vi "Send dashboard control.vi"(7 "timeout":i32=1000, 8 "error in":errorcluster, 10 "Dashboard Control":T1={"Tractive System"=TRUE, "RTD"=TRUE, "AMS error"=TRUE, "IMD error"=TRUE, "Low Voltage"=0.0, "High Voltage"=0.0} {"High Voltage" scale=0.0..10.0; "Low Voltage" scale=0.0..10.0}, 11 "CAN Session In":T2) -> (0 "error out":errorcluster, 3 "CAN Session Out":T2)   [LabVIEW 2016]
uses:
  Program Files (x86)/National Instruments/LabVIEW 2016/examples/robotics/EPOS2 CANOpen Driver/Low Level VIs/Typedefs/CAN Refnum.ctl
  Program Files (x86)/National Instruments/LabVIEW 2016/examples/robotics/EPOS2 CANOpen Driver/Low Level VIs/Typedefs/CAN Session Pointer.ctl
  Program Files (x86)/National Instruments/LabVIEW 2016/examples/robotics/EPOS2 CANOpen Driver/Low Level VIs/Typedefs/CAN Communication References.ctl
  Program Files (x86)/National Instruments/LabVIEW 2016/examples/robotics/EPOS2 CANOpen Driver/Low Level VIs/Typedefs/kill process notifier array.ctl
  Program Files (x86)/National Instruments/LabVIEW 2016/examples/robotics/EPOS2 CANOpen Driver/Low Level VIs/Typedefs/Write Queue.ctl
  Program Files (x86)/National Instruments/LabVIEW 2016/examples/robotics/EPOS2 CANOpen Driver/Low Level VIs/Typedefs/FPGA CAN Frame Cluster.ctl
  Dashboard Control.ctl
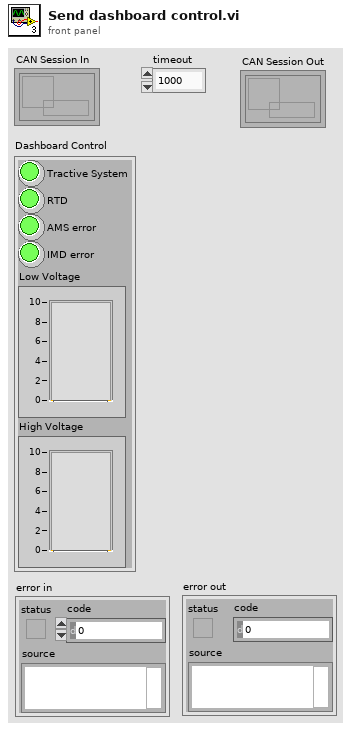
[diagram p1: front panel]
types:
  T1 = typedef "Dashboard Control.ctl" = cluster{"Tractive System":bool, "RTD":bool, "AMS error":bool, "IMD error":bool, "Low Voltage":dbl, "High Voltage":dbl}
  T2 = typedef "CAN Refnum.ctl" = refnum<k1>
  T3 = typedef "FPGA CAN Frame Cluster.ctl" = cluster{"Timestamp":u64, "Identifier":u32, "Type":u8, "InfoA":u8, "InfoB":u8, "DataLength":u8, "Data":u8[]}
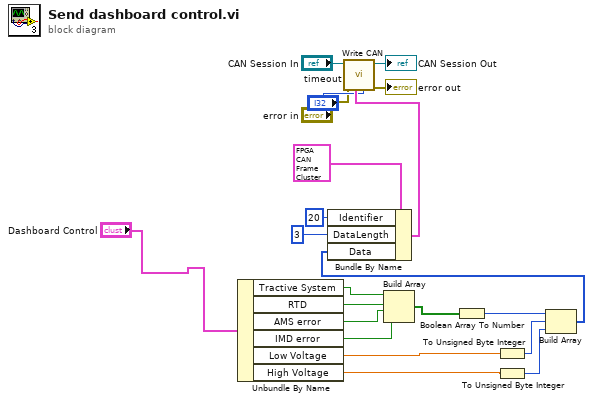
[diagram p0: block diagram]
diagram:
  n1 = Unbundle By Name("Dashboard Control") -> ("Tractive System"=w17:bool, "RTD"=w16:bool, "AMS error"=w15:bool, "IMD error"=w14:bool, "Low Voltage"=w10:dbl, "High Voltage"=w8:dbl)
  n2 = Build Array(w17, w16, w15, w14) -> (w13:bool[])
  n3 = Boolean Array To Number(Boolean array=w13) -> (number=w12:u32)
  n4 = To Unsigned Byte Integer(number=w10) -> (unsigned 8bit integer=w9:u8)
  n5 = To Unsigned Byte Integer(number=w8) -> (unsigned 8bit integer=w7:u8)
  n6 = Build Array(w12, w9, w7) -> (w11:u32[])
  n7 = Bundle By Name(cluster=T3 {"Timestamp"=0, "Identifier"=0, "Type"=0, "InfoA"=0, "InfoB"=0, "DataLength"=0, "Data"=[0, 0, 0, 0, 0, 0, 0, 0]} ("CAN Frame"), "Identifier"=u32 20, "DataLength"=u8 3, "Data"=w11) -> (w20:T3)
  n8 = call "Write CAN.vi"("timeout"="timeout", "CAN Frame"=w20, "error in"="error in", "CAN Session In"="CAN Session In") -> ("error out"=→"error out":errorcluster, "CAN Session Out"=→"CAN Session Out":T2)  [unwired: 6 in]
